vi "Add Step.vi"(8 "error in (no error)":errorcluster, 10 "Step In":refnum<class "Step.lvclass">, 11 "Sequence in":refnum<class "Sequence.lvclass">) -> (0 "error out":errorcluster, 3 "Sequence out":refnum<class "Sequence.lvclass">)   [LabVIEW 2015, in "Mediator.lvlib" / "Sequence.lvclass"]
doc: "This adds a step to the Sequence."
uses:
  Sequence.lvclass
  Step/Step.lvclass
  Sequence.lvclass/Sequence.ctl
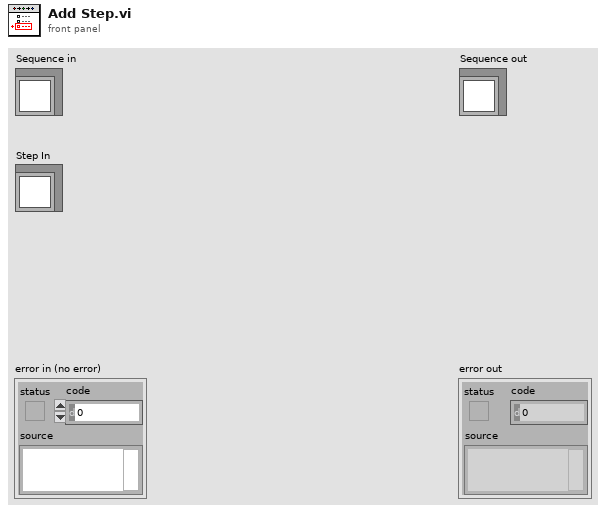
[diagram p1: front panel]
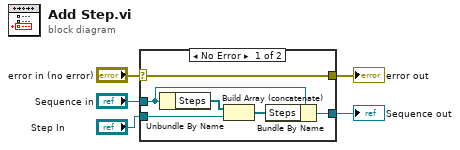
[diagram p0: block diagram]
diagram:
  n1 = case shown="No Error" "error in (no error)" {
    selector: "error in (no error)" -> [w11 w13]
    tunnel: [w11 w13] -> w4
    tunnel: [w6 w12] -> w2
    tunnel: "Sequence in" -> [w7 w12]
    tunnel: "Step In" -> [w9 _]
    frame No Error {
      n2 = Unbundle By Name(w7) -> ("Steps"=w10:refnum<class "Step.lvclass">[])
      n3 = Build Array (concatenate)(w10, w9) -> (w8:refnum<class "Step.lvclass">[])
      n4 = Bundle By Name(cluster=w7, "Steps"=w8) -> (w6:refnum<class "Sequence.lvclass">)
    }
    frame Error {
    }
  }
  "error out" <- w4
  "Sequence out" <- w2
